vi "logrecordstring.vi"(7 "logsetting":enum16{"error", "info", "debug"}(ring), 8 "error in":errorcluster, 9 "logtype":enum16{"error", "info", "debug"}(ring), 10 "LogPath":path, 11 "Msg":string) -> (0 "error out":errorcluster)   [LabVIEW 2011]
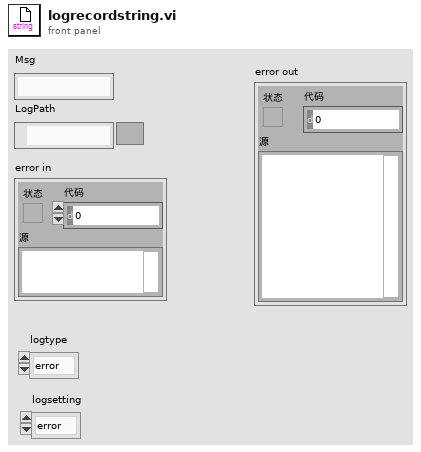
[diagram p1: front panel]
types:
  T1 = enum16{"open", "replace", "create", "open or create", "replace or create", "replace or create with confirmation"}
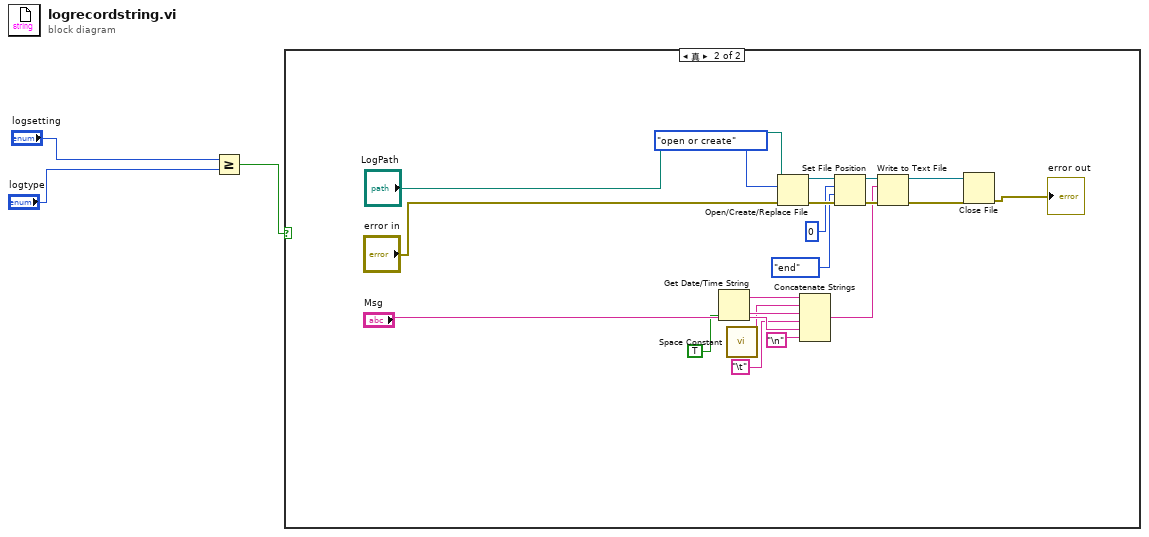
[diagram p0: block diagram]
diagram:
  n1 = Greater Or Equal?(x="logsetting", y="logtype") -> (x >= y?=w1:bool)
  n2 = case shown="真" w1 {
    frame False {
    }
    frame True {
      n3 = Get Date/Time String(want seconds? (F)=TRUE ("需要秒？(F)")) -> (date string=w8:string, time string=w10:string)  [unwired: 2 in]
      n4 = call <vilib>:"Space Constant.vi"() -> ("String"=w9:string)
      n5 = Open/Create/Replace File(file path (use dialog)="LogPath", error in="error in", operation (0:open)=T1."open or create" ("操作(0:open)")) -> (refnum out=w4:refnum<file>, error out=w15:errorcluster)  [unwired: 3 in, 1 out]
      n6 = Concatenate Strings(w8, w9, w10, "\t", "Msg", "\n") -> (w13:string)
      n7 = Set File Position(offset (in bytes) (0)=i64 0 ("偏移量（字节）（0）"), refnum=w4, from (0:start)=enum16{"start", "end", "current"}."end" ("自（0:起始）"), error in=w15) -> (refnum out=w6:refnum<file>, error out=w16:errorcluster)
      n8 = Write to Text File(file (use dialog)=w6, text=w13, error in=w16) -> (refnum out=w18:refnum<file>, error out=w19:errorcluster)  [unwired: 1 in, 1 out]
      n9 = Close File(refnum=w18, error in=w19) -> (error out=→"error out":errorcluster)  [unwired: 1 out]
    }
  }
